vi "Golden Section Inner Part (VI).vi"(0 "a (start)":dbl format="%.2f", 1 "f(x)":T1, 2 "accuracy":dbl format="%.2f", 5 "b (start)":dbl format="%.2f", 7 "c (start)":dbl format="%.2f", 11 "error in":i32, 12 "data":variant, 13 "case":bool, 14 "sign":i32(ring) items=["y=f(x)", "y=-f(x)"]) -> (4 "minimum":dbl format="%.2f", 6 "f(minimum)":dbl format="%.2f", 15 "error out":i32)   [LabVIEW 2014, in "NI_Gmath.lvlib"]
uses:
  NI_Gmath.lvlib
  functionRefnum.ctl
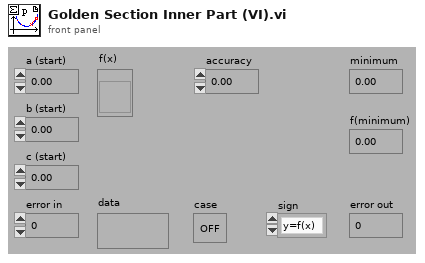
[diagram p1: front panel]
types:
  T1 = typedef "NI_Gmath.lvlib/functionRefnum.ctl" = refnum<vi>
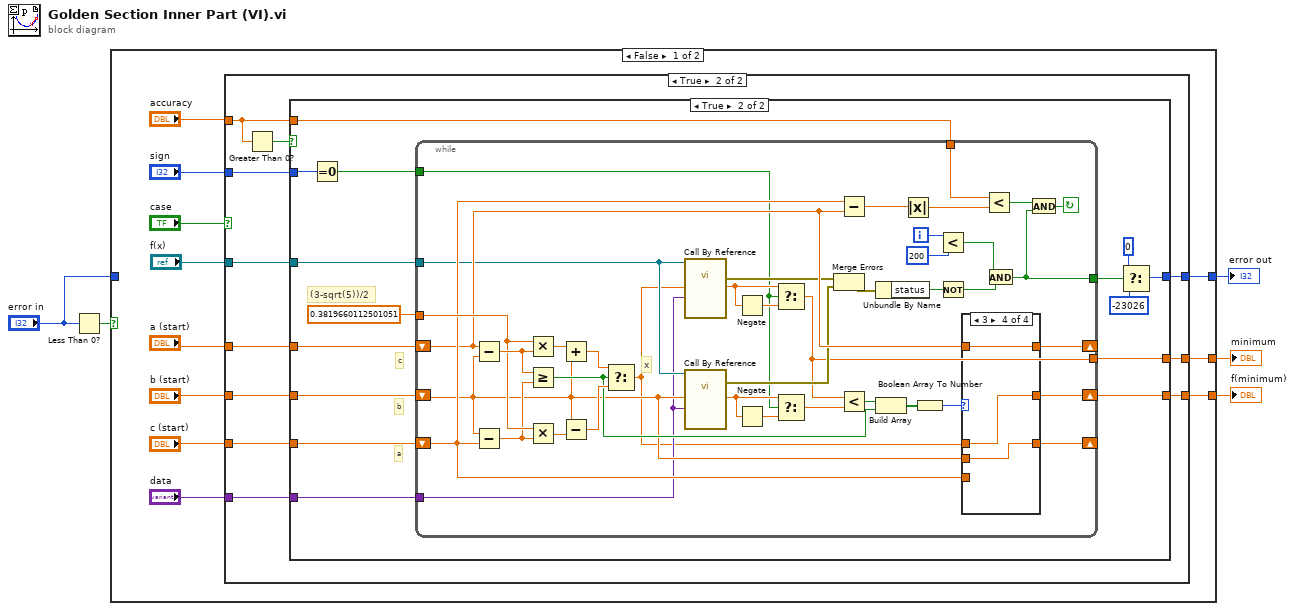
[diagram p0: block diagram]
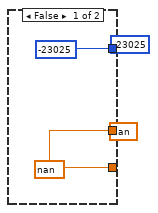
[diagram p2: hidden frame]
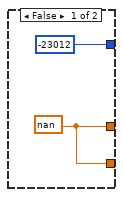
[diagram p3: hidden frame]
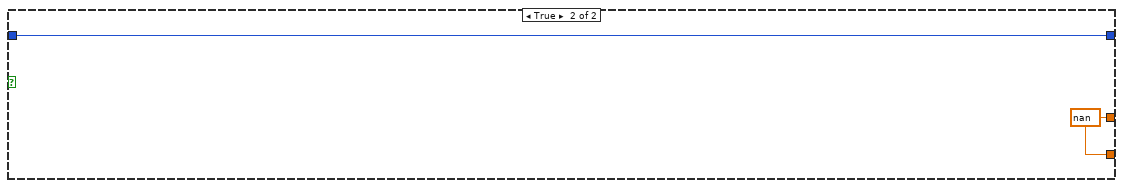
[diagram p7: hidden frame]
diagram:
  n1 = Less Than 0?(x="error in") -> (x < 0?=w2:bool)
  n2 = case shown="False" w2 {
    tunnel: [w8 w101] -> w5
    tunnel: [w10 w100] -> w4
    tunnel: [w9 w100] -> w3
    tunnel: "error in" -> [_ w101]
    frame False {
      n3 = case shown="True" "case" {
        tunnel: "c (start)" -> [_ w29]
        tunnel: "b (start)" -> [_ w28]
        tunnel: "a (start)" -> [_ w27]
        tunnel: "accuracy" -> [_ w25]
        tunnel: "f(x)" -> [_ w24]
        tunnel: "data" -> [_ w23]
        tunnel: [w18 w20] -> w10
        tunnel: [w18 w22] -> w9
        tunnel: [-23025 w21] -> w8
        tunnel: "sign" -> [_ w19]
        frame False {
          w18 = nan
          (unwired) -23025
          (unwired) nan
        }
        frame True {
          n4 = Greater Than 0?(x=w25) -> (x > 0?=w26:bool)
          n5 = case shown="True" w26 {
            tunnel: [w30 w40] -> w22
            tunnel: w27 -> [_ w46]
            tunnel: w28 -> [_ w45]
            tunnel: w29 -> [_ w44]
            tunnel: w25 -> [_ w43]
            tunnel: [-23012 w36] -> w21
            tunnel: w24 -> [_ w42]
            tunnel: w23 -> [_ w41]
            tunnel: [w30 w35] -> w20
            tunnel: w19 -> [_ w34]
            frame False {
              w30 = nan
            }
            frame True {
              # "(3-sqrt(5))/2"
              # "a"
              # "b"
              # "c"
              n6 = Equal To 0?(x=w34) -> (x = 0?=w33:bool)
              n7 = while {
                tunnel: [w58] -> w39
                tunnel: w43 -> [w85]
                tunnel: 0.3819660112501051 ("x*y") -> [w78]
                shift-left: w46 -> [w68]
                shift-right: [w65] -> _
                shift-left: w45 -> [w63]
                shift-right: [w66] -> w35
                shift-left: w44 -> [w69]
                shift-right: [w67] -> _
                tunnel: w42 -> [w64]
                tunnel: w41 -> [w62]
                tunnel: [w53] -> w40
                tunnel: w33 -> [w47]
                i -> [w84]
                stop <- w81 continue-if-true
                # "x"
                n8 = Subtract(x=w68, y=w63) -> (x-y=w80:dbl)
                n9 = Subtract(x=w63, y=w69) -> (x-y=w77:dbl)
                n10 = Multiply(x=w78, y=w80) -> (x*y=w79:dbl)
                n11 = Greater Or Equal?(x=w80, y=w77) -> (x >= y?=w72:bool)
                n12 = Multiply(x=w78, y=w77) -> (x*y=w76:dbl)
                n13 = Add(x=w79, y=w63) -> (x+y=w74:dbl)
                n14 = Subtract(x=w63, y=w76) -> (x-y=w75:dbl)
                n15 = Select(t=w74, s=w72, f=w75) -> (s? t:f=w56:dbl)
                n16 = call-by-ref "?"(reference=w64, "Variant"=w62, "x"=w56) -> (error out=w55:errorcluster, "f(x)"=w51:dbl)  [unwired: 4 in, 1 out]
                n17 = call-by-ref "?"(reference=w64, "Variant"=w62, "x"=w63) -> (error out=w54:errorcluster, "f(x)"=w48:dbl)  [unwired: 4 in, 1 out]
                n18 = Negate(x=w51) -> (-x=w52:dbl)
                n19 = Negate(x=w48) -> (-x=w50:dbl)
                n20 = Select(t=w51, s=w47, f=w52) -> (s? t:f=w53:dbl)
                n21 = Select(t=w48, s=w47, f=w50) -> (s? t:f=w49:dbl)
                n22 = Merge Errors(w55, w54) -> (w61:errorcluster)
                n23 = Subtract(x=w69, y=w68) -> (x-y=w87:dbl)
                n24 = Less?(x=w53, y=w49) -> (x < y?=w73:bool)
                n25 = Unbundle By Name(w61) -> ("status"=w59:bool)
                n26 = Build Array(w73, w72) -> (w71:bool[])
                n27 = Absolute Value(x=w87) -> (abs(x)=w86:dbl)
                n28 = Boolean Array To Number(Boolean array=w71) -> (number=w70:u32)
                n29 = Less?(x=w84, y=200) -> (x < y?=w60:bool)
                n30 = Not(x=w59) -> (.not. x?=w57:bool)
                n31 = case shown="3" w70 {
                  tunnel: w69 -> [_ w93 w95 _]
                  tunnel: w63 -> [w89 w91 w96 w99]
                  tunnel: w68 -> [w88 _ _ w98]
                  tunnel: w56 -> [w90 w92 w94 w97]
                  tunnel: [w90 w93 w95 w99] -> w67
                  tunnel: [w89 w92 w96 w97] -> w66
                  tunnel: [w88 w91 w94 w98] -> w65
                  frame 0, Default {
                  }
                  frame 1 {
                  }
                  frame 2 {
                  }
                  frame 3 {
                  }
                }
                n32 = Less?(x=w85, y=w86) -> (x < y?=w82:bool)
                n33 = And(x=w60, y=w57) -> (x .and. y?=w58:bool)
                n34 = And(x=w82, y=w58) -> (x .and. y?=w81:bool)
              }
              n35 = Select(t=0, s=w39, f=-23026) -> (s? t:f=w36:i32)
            }
          }
        }
      }
    }
    frame True {
      w100 = nan ("result")
    }
  }
  "error out" <- w5
  "f(minimum)" <- w4
  "minimum" <- w3
